vi "GUI.SelectOPCTags.vi"(7 "Mode":T1, 8 "error in":errorcluster, 11 "Section Ptr":T2 format="%.0x") -> (0 "error out":errorcluster)   [LabVIEW 2019, in "OPC UA Client Addon System Explorer.lvlib"]
uses:
  OPC UA Client Addon System Explorer.lvlib
  <vilib>/NI VeriStand/Custom Device API/Custom Device Item Ref.ctl
  Types/Tag.SelectionMode.ctl
  <vilib>/NI/AMC/Read Termination Message.vi
  <vilib>/NI/AMC/Create Single Message.vi
  <vilib>/NI/AMC/Update Message Routing Info.vi
  <vilib>/NI/AMC/Create Multiple Messages.vi
  <vilib>/NI/AMC/Globals.vi
  Addon Shared/Constants.vi
  <vilib>/NI VeriStand/Custom Device Tools/Custom Device Utility Library/NI VeriStand - Search for All Items by GUID.vi
  <vilib>/NI VeriStand/Custom Device API/NI VeriStand - Get Item Property.vi
  <vilib>/NI VeriStand/Custom Device API/Get Item Property (String).vi
  <vilib>/NI VeriStand/Custom Device API/Get Item Property (U16).vi
  <vilib>/NI VeriStand/Custom Device API/Get Item Property (Dependent File).vi
  <vilib>/NI VeriStand/Custom Device API/NI VeriStand - Set Item Property.vi
  <vilib>/NI VeriStand/Custom Device API/Set Item Property (String).vi
  <vilib>/NI VeriStand/Custom Device API/Set Item Property (U16).vi
  <vilib>/Utility/libraryn.llb/Get File Extension.vi
  <vilib>/Utility/MD5Checksum.llb/MD5Checksum File.vi
  <vilib>/NI VeriStand/Custom Device API/Set Item Property (Dependent File).vi
  <vilib>/Utility/libraryn.llb/Check if File or Folder Exists.vi
  <vilib>/NI VeriStand/Custom Device API/NI VeriStand - Remove Item Property.vi
  <vilib>/NI/AMC/Send Message.vi
  <vilib>/NI/AMC/AMC.lvlib
  <vilib>/NI VeriStand/Custom Device API/Custom Device API.lvlib
  <vilib>/NI VeriStand/Custom Device Tools/Custom Device Utility Library/Custom Device Utility Library.lvlib
  Addon Shared/OPC UA Client Addon Shared.lvlib
panel:
  in  "OK":bool
  in  "Cancel":bool
  in  "Tree":string(tree)
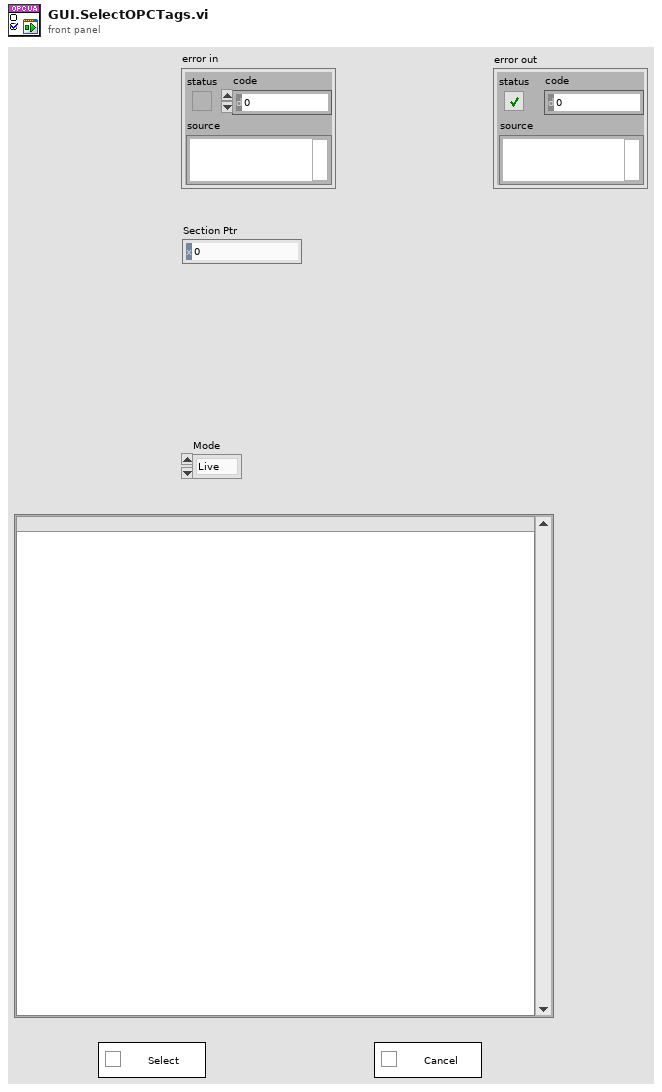
[diagram p1: front panel]
types:
  T1 = typedef "OPC UA Client Addon System Explorer.lvlib/Tag.SelectionMode.ctl" = enum8{"Live", "Offline"}
  T2 = typedef "Custom Device API.lvlib/Custom Device Item Ref.ctl" = u64
  T3 = cluster{"name":string, "node type":enum32{"Other", "Folder", "Item/Property"}, "DataType":u32, "access":enum16{"Null", "Read", "Write", "Read&Write"}, "description":string}
  T4 = typedef "AMC.lvlib/Message Queue.ctl" = refnum<queue>
  T5 = typedef "Custom Device API.lvlib/Custom Device Item Info.ctl" = cluster{"Name":string, "Is Channel":bool, "GUID":string, "Is Waveform":bool}
  T6 = typedef "OPC UA Client Addon Shared.lvlib/OPCConnection.Properties.ctl" = cluster{"Server IP Address":string, "Server Port":u16, "Message Mode":enum16{"None", "Sign", "Sign and Encrypt"}, "Security":enum16{"Basic256", "Basic128Rsa15"}, "User Name":string, "Password":string, "Client Certificate":path, "Server Certificate":path, "Server Certificate (RT)":path, "Client Certificate (RT)":path}
  T7 = typedef "LVPoint32TypeDef.ctl" = cluster{"Horizontal":i32, "Vertical":i32}
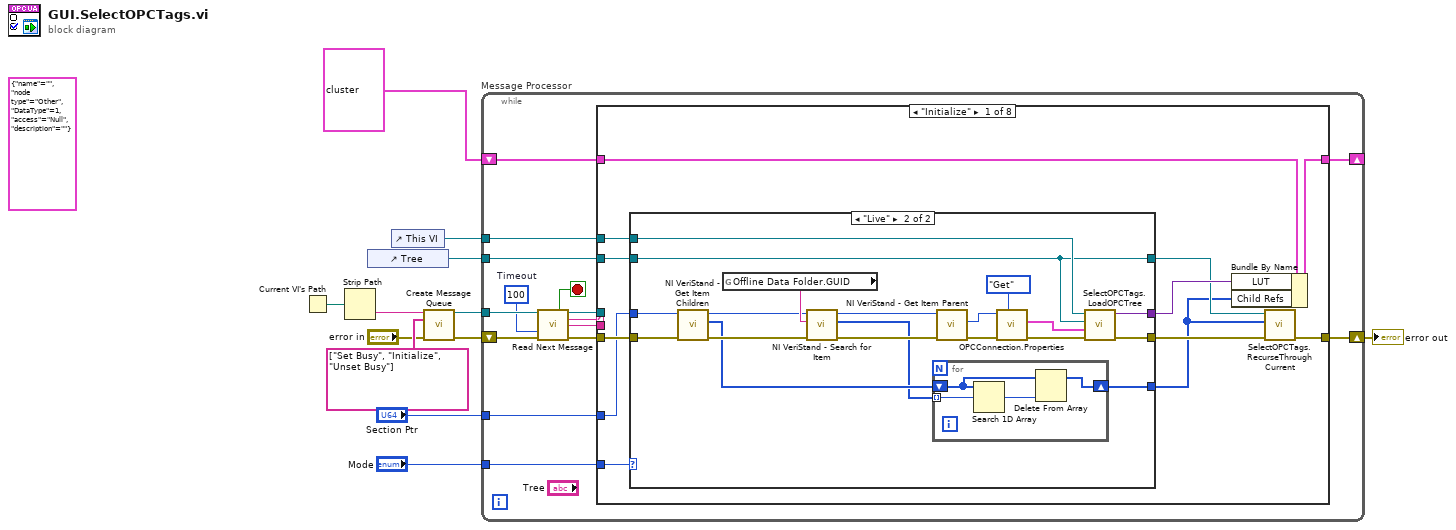
[diagram p0: block diagram]
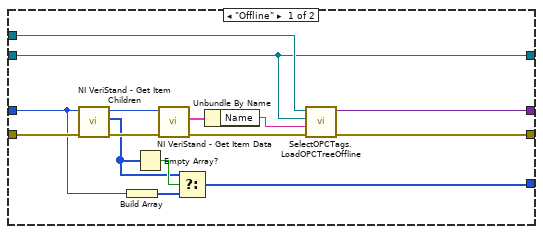
[diagram p2: hidden frame]
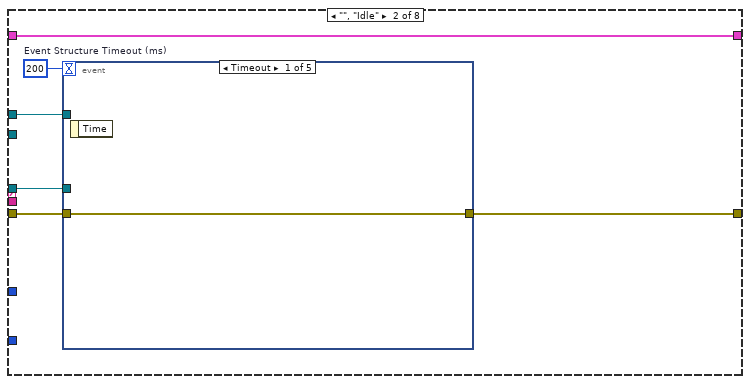
[diagram p3: hidden frame]
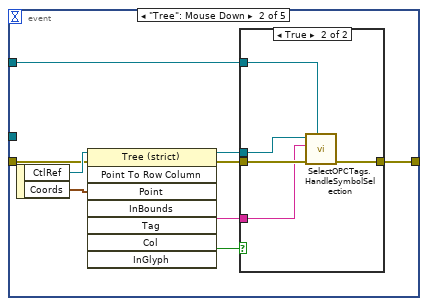
[diagram p4: hidden frame]
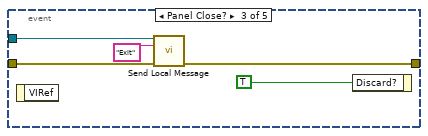
[diagram p6: hidden frame]
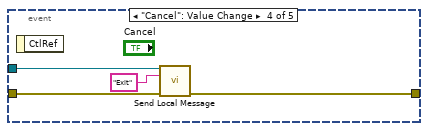
[diagram p7: hidden frame]
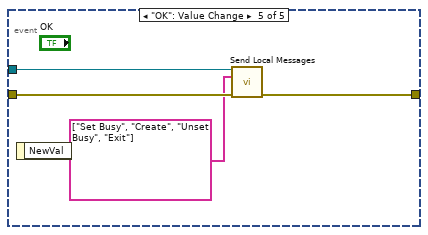
[diagram p8: hidden frame]
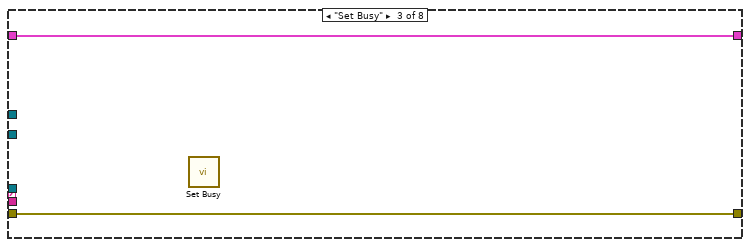
[diagram p9: hidden frame]
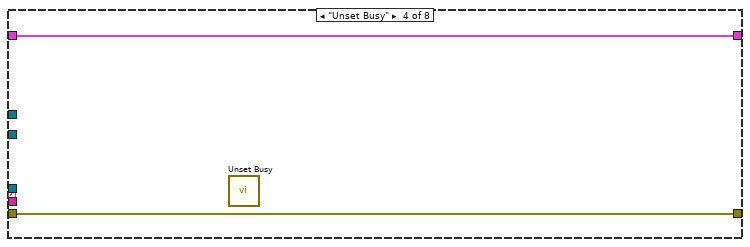
[diagram p10: hidden frame]
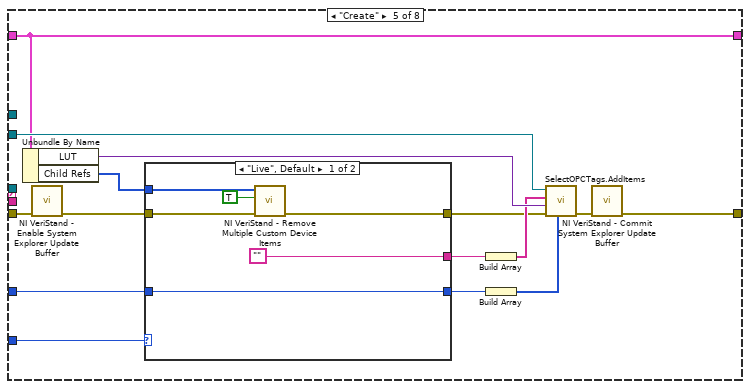
[diagram p11: hidden frame]
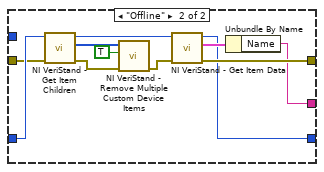
[diagram p12: hidden frame]
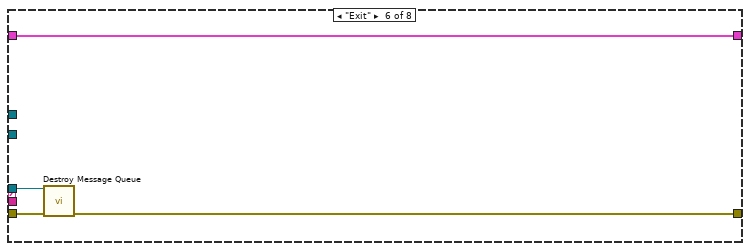
[diagram p13: hidden frame]
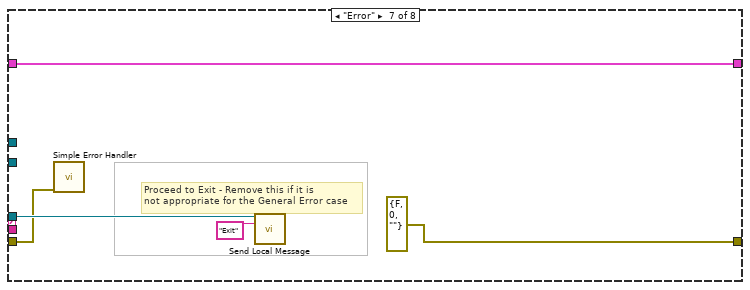
[diagram p14: hidden frame]
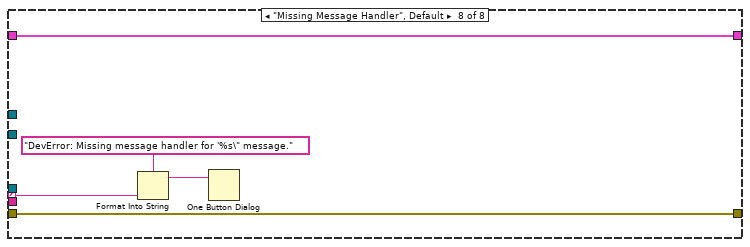
[diagram p15: hidden frame]
diagram:
  (unwired) T3 {"name"="", "node type"=enum."Other", "DataType"=1, "access"=enum."Null", "description"=""} ("node attribute")
  n1 = Current VI's Path() -> (path=w8:path)
  n2 = Strip Path(path=w8) -> (name=w11:string)  [unwired: 1 out]
  n3 = control-ref of="Tree"() -> (w5:refnum<vi>)
  n4 = control-ref of="This VI"() -> (w4:refnum<vi>)
  n5 = call <vilib>:"Create Message Queue.vi"("message queue name"=w11, "initial message names"=string[] ["Set Busy", "Initialize", "Unset Busy"], "error in"="error in") -> ("message queue out"=w10:T4, "error out"=w9:errorcluster)  [unwired: 11 in]
  n6 = while "Message Processor" {
    shift-left: w9 -> [w23]
    shift-right: [w27] -> w6
    tunnel: w10 -> [w24]
    tunnel: w5 -> [w18]
    tunnel: w4 -> [w17]
    shift-right: [w16] -> _
    shift-left: cluster{"LUT":variant, "Child Refs":T2[]} {"LUT"=variant, "Child Refs"=[]} -> [w15]
    tunnel: "Section Ptr" -> [w14]
    tunnel: "Mode" -> [w13]
    stop <- w26 stop-if-true
    w19 = 100  # Timeout
    n7 = call <vilib>:"Read Next Message.vi"("message queue in"=w24, "timeout (1 ms)"=w19, "error in"=w23) -> ("exit process?"=w26:bool, "message queue out"=w25:T4, "message name"=w21:string, "message value"=w20:string, "error out"=w22:errorcluster)  [unwired: 5 in, 3 out]
    n8 = case shown="\"Initialize\"" w21 {
      selector: w21 -> [_ _ _ _ _ _ _ w161]
      tunnel: w25 -> [_ w82 _ _ _ w151 w156 _]
      tunnel: w22 -> [w35 w81 w113 w115 w126 w152 w154 w162]
      tunnel: [w30 w80 w113 w115 w124 w150 errorcluster {"status"=FALSE, "code"=0, "source"=""} ("error out") w162] -> w27
      tunnel: w20 -> [_ _ _ _ _ _ _ _]
      tunnel: w18 -> [w39 _ _ _ w131 _ _ _]
      tunnel: w17 -> [w38 w78 _ _ _ _ _ _]
      tunnel: [w36 w79 w114 w116 w129 w149 w153 w158] -> w16
      tunnel: w15 -> [w37 w79 w114 w116 w129 w149 w153 w158]
      tunnel: w14 -> [w34 _ _ _ w119 _ _ _]
      tunnel: w13 -> [w32 _ _ _ w123 _ _ _]
      frame "Initialize" {
        n9 = case shown="\"Live\"" w32 {
          tunnel: [w54 w73] -> w31
          tunnel: w39 -> [w48 w65]
          tunnel: w38 -> [w53 w72]
          tunnel: w35 -> [w47 w60]
          tunnel: w34 -> [w40 w61]
          tunnel: [w52 w70] -> w33
          tunnel: [w48 w65] -> w29
          tunnel: [w41 w55] -> w28
          frame "Offline" {
            n10 = call <vilib>:"NI VeriStand - Get Item Children.vi"("error in (no error)"=w47, "Item Ref in"=w40) -> ("error out"=w46:errorcluster, "Child Refs"=w43:T2[], "Item Ref out"=w45:T2)  [unwired: 6 in, 1 out]
            n11 = Build Array(w40) -> (w42:T2[])
            n12 = Empty Array?(array=w43) -> (empty?=w44:bool)
            n13 = call <vilib>:"NI VeriStand - Get Item Data.vi"("error in (no error)"=w46, "Item Ref in"=w45) -> ("error out"=w50:errorcluster, "Item Info"=w51:T5)  [unwired: 8 out]
            n14 = Select(t=w43, s=w44, f=w42) -> (s? t:f=w41:T2[])
            n15 = Unbundle By Name(w51) -> ("Name"=w49:string)
            n16 = call "SelectOPCTags.LoadOPCTreeOffline.vi"("error in"=w50, "Channel"=w49, "Tree"=w48, "VI in"=w53) -> ("error out"=w54:errorcluster, "LUT"=w52:variant)  [unwired: 6 in]
          }
          frame "Live" {
            n17 = call <vilib>:"NI VeriStand - Get Item Children.vi"("error in (no error)"=w60, "Item Ref in"=w61) -> ("error out"=w59:errorcluster, "Child Refs"=w57:T2[], "Item Ref out"=w58:T2)  [unwired: 6 in, 1 out]
            n18 = global read "Constants.vi" "Offline Data Folder.GUID"() -> (w62:string)
            n19 = call-poly <vilib>:"NI VeriStand - Search for Item.vi"("error in"=w59, "Item GUID"=w62, "Section Ref in"=w58) -> ("error out"=w64:errorcluster, "Item Refs"=w56:T2[], "Section Ref out"=w63:T2)  [unwired: 5 in, 1 out]
            n20 = for {
              shift-right: [w74] -> w55
              shift-left: w57 -> [w76]
              tunnel: w56 -> [w77] mode=indexing
              n21 = Search 1D Array(1D array=w76, element=w77) -> (index of element=w75:i32)  [unwired: 1 in]
              n22 = Delete From Array(array=w76, index=w75) -> (array with subset deleted=w74:T2[])  [unwired: 1 in, 1 out]
            }
            n23 = call <vilib>:"NI VeriStand - Get Item Parent.vi"("error in (no error)"=w64, "Item Ref in"=w63) -> ("error out"=w67:errorcluster, "Parent Ref"=w66:T2)  [unwired: 6 in, 2 out]
            n24 = call "OPCConnection.Properties.vi"("Action"=enum8{"Get", "Set"}."Get", "error in (no error)"=w67, "Item Ref in"=w66) -> ("error out"=w71:errorcluster, "Connection.Properties"=w69:T6)  [unwired: 6 in, 1 out]
            n25 = call "SelectOPCTags.LoadOPCTree.vi"("error in (no error)"=w71, "Connection.Properties"=w69, "Tree"=w65, "VI in"=w72) -> ("error out"=w73:errorcluster, "LUT"=w70:variant)  [unwired: 6 in]
          }
        }
        n26 = Bundle By Name(cluster=w37, "LUT"=w33, "Child Refs"=w28) -> (w36:cluster{"LUT":variant, "Child Refs":T2[]})
        n27 = call "SelectOPCTags.RecurseThroughCurrent.vi"("error in (no error)"=w31, "Node Pointer"=w28, "Tree"=w29) -> ("error out"=w30:errorcluster)  [unwired: 7 in, 1 out]
      }
      frame "", "Idle" {
        w83 = 200  # Event Structure Timeout (ms)
        n28 = event shown="[0] Timeout" {
          selector: _ -> [_ _ _ _ _]
          dyn-events: _ -> [_ _ _ _ _]
          timeout: w83 -> [_ _ _ _ _]
          tunnel: w82 -> [_ _ w103 w107 w111]
          tunnel: w81 -> [w84 w91 w102 w105 w112]
          tunnel: [w84 w86 w101 w106 w110] -> w80
          tunnel: w78 -> [_ w85 _ _ _]
          event Timeout {
            n29 = event-data() -> ()  [unwired: 2 out]
          }
          event "Tree": Mouse Down {
            n30 = event-data() -> ("CtlRef"=w93:refnum<vi>, "Coords"=w92:T7)  [unwired: 1 out]
            n31 = invoke class="Tree (strict)" method="Point To Row Column"(reference=w93, error in=w91, "Point"=w92) -> (reference out=w87:refnum<vi>, error out=w89:errorcluster, "Tag"=w88:string, "InGlyph"=w90:bool)  [unwired: 5 in, 4 out]
            n32 = case shown="True" w90 {
              tunnel: w89 -> [w94 w99]
              tunnel: w88 -> [_ w97]
              tunnel: w87 -> [_ w98]
              tunnel: [w94 w96] -> w86
              tunnel: w85 -> [_ w95]
              frame False {
              }
              frame True {
                n33 = call "SelectOPCTags.HandleSymbolSelection.vi"("This VI"=w95, "error in"=w99, "Tag"=w97, "CtlRef"=w98) -> ("error out"=w96:errorcluster)  [unwired: 7 in]
              }
            }
          }
          event Panel Close? {
            n34 = event-data() -> ()  [unwired: 2 out]
            n35 = call <vilib>:"Send Local Message.vi"("message queue in"=w103, "message name"="Exit", "error in"=w102) -> ("error out"=w101:errorcluster)  [unwired: 10 in, 2 out]
            n36 = event-data("Discard?"=TRUE) -> ()  [unwired: 1 in, 1 out]
          }
          event "Cancel": Value Change {
            n37 = event-data() -> ()  [unwired: 2 out]
            n38 = call <vilib>:"Send Local Message.vi"("message queue in"=w107, "message name"="Exit", "error in"=w105) -> ("error out"=w106:errorcluster)  [unwired: 10 in, 2 out]
          }
          event "OK": Value Change {
            n39 = event-data() -> ()  [unwired: 2 out]
            n40 = call <vilib>:"Send Local Messages.vi"("message queue in"=w111, "message names"=string[] ["Set Busy", "Create", "Unset Busy", "Exit"], "error in"=w112) -> ("error out"=w110:errorcluster)  [unwired: 10 in, 2 out]
          }
        }
      }
      frame "Set Busy" {
        n41 = call <vilib>:"Set Busy.vi"() -> ()  [unwired: 10 in, 2 out]
      }
      frame "Unset Busy" {
        n42 = call <vilib>:"Unset Busy.vi"() -> ()  [unwired: 11 in, 1 out]
      }
      frame "Create" {
        n43 = Unbundle By Name(w129) -> ("LUT"=w128:variant, "Child Refs"=w117:T2[])
        n44 = call <vilib>:"NI VeriStand - Enable System Explorer Update Buffer.vi"("error in (no error)"=w126) -> ("error out"=w118:errorcluster)  [unwired: 10 in]
        n45 = case shown="\"Live\", Default" w123 {
          tunnel: w119 -> [w136 w143]
          tunnel: [w136 w146] -> w122
          tunnel: w118 -> [w134 w141]
          tunnel: [w133 w147] -> w121
          tunnel: ["" w145] -> w120
          tunnel: w117 -> [w132 _]
          frame "Live", Default {
            n46 = call <vilib>:"NI VeriStand - Remove Multiple Custom Device Items.vi"("error in (no error)"=w134, "Force Delete (F)"=TRUE, "Item Refs in"=w132) -> ("error out"=w133:errorcluster)  [unwired: 7 in, 1 out]
          }
          frame "Offline" {
            n47 = call <vilib>:"NI VeriStand - Get Item Children.vi"("error in (no error)"=w141, "Item Ref in"=w143) -> ("error out"=w140:errorcluster, "Child Refs"=w139:T2[], "Item Ref out"=w142:T2)  [unwired: 6 in, 1 out]
            n48 = call <vilib>:"NI VeriStand - Remove Multiple Custom Device Items.vi"("error in (no error)"=w140, "Force Delete (F)"=TRUE, "Item Refs in"=w139) -> ("error out"=w138:errorcluster)  [unwired: 7 in, 1 out]
            n49 = call <vilib>:"NI VeriStand - Get Item Data.vi"("error in (no error)"=w138, "Item Ref in"=w142) -> ("error out"=w147:errorcluster, "Item Info"=w148:T5, "Item Ref out"=w146:T2)  [unwired: 7 out]
            n50 = Unbundle By Name(w148) -> ("Name"=w145:string)
          }
        }
        n51 = Build Array(w120) -> (w127:string[])
        n52 = Build Array(w122) -> (w130:T2[])
        n53 = call "SelectOPCTags.AddItems.vi"("VS Refs"=w130, "error in (no error)"=w121, "LUT"=w128, "Items"=w127, "TreeControl in"=w131) -> ("error out"=w125:errorcluster)  [unwired: 6 in]
        n54 = call <vilib>:"NI VeriStand - Commit System Explorer Update Buffer.vi"("error in (no error)"=w125) -> ("error out"=w124:errorcluster)  [unwired: 10 in]
      }
      frame "Exit" {
        n55 = call <vilib>:"Destroy Message Queue.vi"("message queue in"=w151, "error in"=w152) -> ("error out"=w150:errorcluster)  [unwired: 11 in, 2 out]
      }
      frame "Error" {
        # "Proceed to Exit - Remove this if it is\nnot appropriate for the General Error case"
        n56 = call <vilib>:"Simple Error Handler.vi"("error in (no error)"=w154) -> ()  [unwired: 1 in, 8 out]
        n57 = call <vilib>:"Send Local Message.vi"("message queue in"=w156, "message name"="Exit") -> ()  [unwired: 11 in, 3 out]
      }
      frame "Missing Message Handler", Default {
        n58 = Format Into String(format string="DevError: Missing message handler for '%s\" message." ("message"), w161) -> (resulting string=w159:string)  [unwired: 2 in, 1 out]
        n59 = One Button Dialog(message=w159) -> ()  [unwired: 2 out]
      }
    }
  }
  "error out" <- w6
